vi "dotNetExceptionWrapper.vi"(3 "error in":errorcluster) -> (1 "error out":errorcluster)   [LabVIEW 2011, in "Konvolucio MCAN120803.lvlib"]
uses:
  <instrlib>/Konvolucio MCAN120803/Konvolucio MCAN120803.lvlib
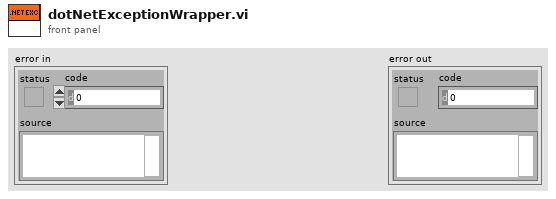
[diagram p1: front panel]
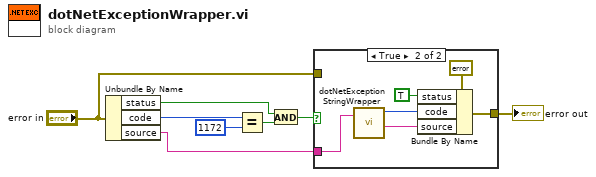
[diagram p0: block diagram]
diagram:
  n1 = Unbundle By Name("error in") -> ("status"=w5:bool, "code"=w8:i32, "source"=w3:string)
  n2 = Equal?(x=w8, y=1172) -> (x = y?=w6:bool)
  n3 = And(x=w5, y=w6) -> (x .and. y?=w4:bool)
  n4 = case shown="True" w4 {
    tunnel: w3 -> [_ w13]
    tunnel: "error in" -> [w9 _]
    tunnel: [w9 w15] -> w2
    frame False {
    }
    frame True {
      n5 = call <instrlib>:"dotNetExceptionStringWrapper.vi"("ExceptionIn"=w13) -> ("Code"=w12:i32, "ExceptionOut"=w11:string)  [unwired: 3 in]
      n6 = Bundle By Name(cluster=errorcluster {"status"=FALSE, "code"=0, "source"=""} ("error IO"), "status"=TRUE, "code"=w12, "source"=w11) -> (w15:errorcluster)
    }
  }
  "error out" <- w2
